vi "CCSaveQueryAsDcmFile.vi"(8 "error in (no error)":errorcluster, 9 "patientID":string="C:\\Users\\Simon\\Dropbox\\Medimatic\\ProjectVerLV2011\\tmp.dcm", 10 "index":i32, 11 "Find":refnum<k24>) -> (0 "error out":errorcluster)   [LabVIEW 2013, in "main.lvlib" / "ClearCanvasLibrary.lvlib"]
uses:
  ClearCanvasLibrary.lvlib
  C:/Users/Simon/SkyDrive/LabView/2013/DM2020/DICOM/ClearCanvasNewBuild/ClearCanvas.Dicom.dll
  ClearCanvasNewBuild/ClearCanvas.Dicom.dll
  Globals/DataPathGlobalVariable.vi
  main.lvlib
  <userlib>/_OpenG.lib/file/file.llb/File Exists - Scalar__ogtk.vi
panel:
  out "DumpString":string
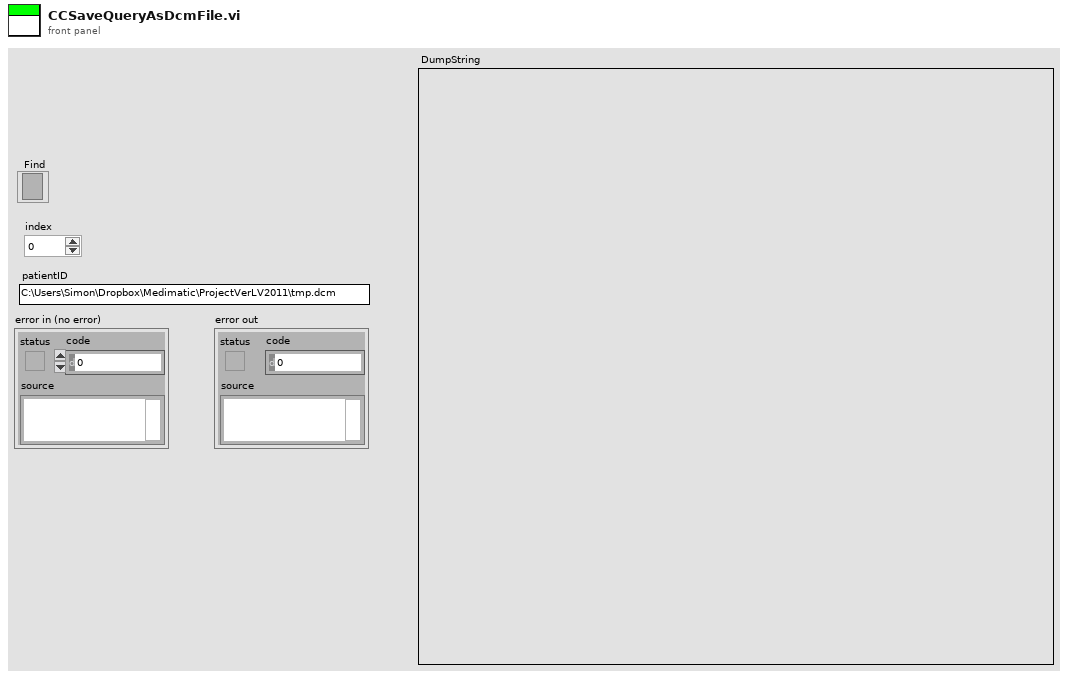
[diagram p1: front panel]
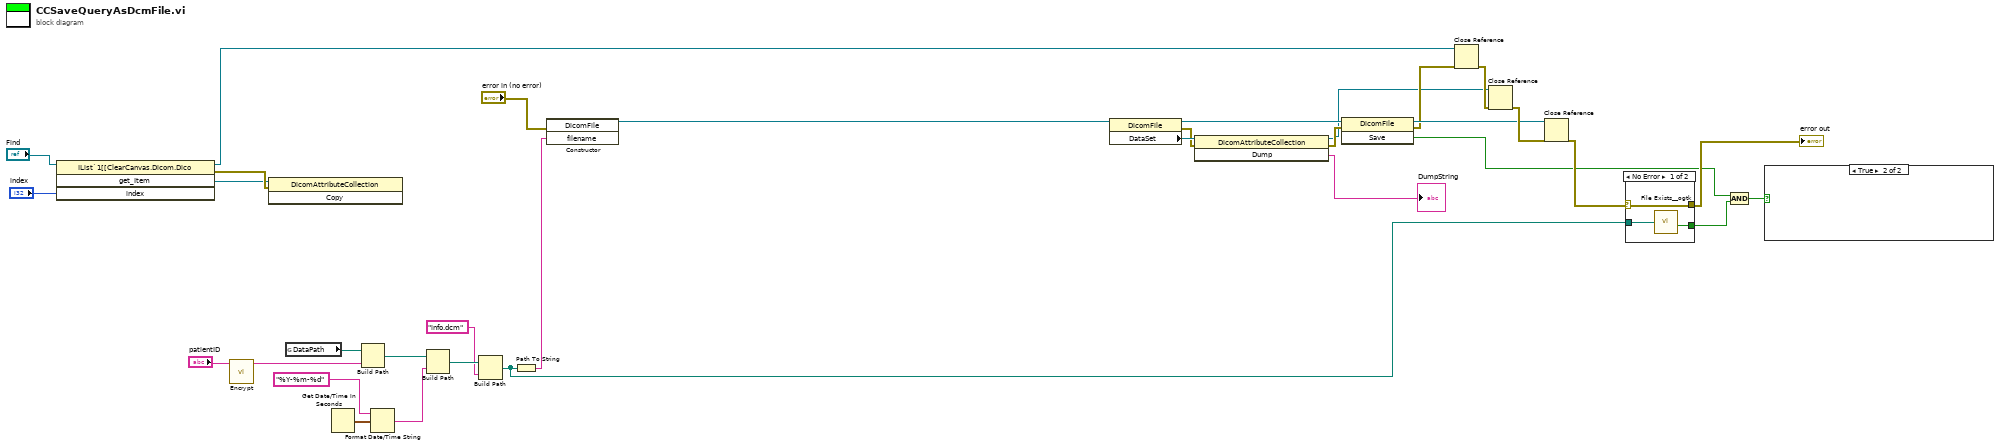
[diagram p0: block diagram]
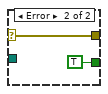
[diagram p2: hidden frame]
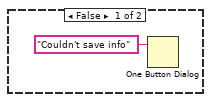
[diagram p3: hidden frame]
diagram:
  n1 = invoke class="IList`1[[ClearCanvas.Dicom.Dico" method="get_Item"(reference="Find", "index"="index") -> (reference out=w2:refnum<k24>, error out=w15:errorcluster, "get_Item"=w1:refnum<k24>)  [unwired: 2 in, 1 out]
  n2 = call "Encrypt.vi"("Input"="patientID") -> ("Output"=w21:string)  [unwired: 10 in]
  n3 = invoke class="DicomAttributeCollection" method="Copy"(reference=w1, error in=w15) -> ()  [unwired: 1 in, 3 out]
  n4 = global read "DataPathGlobalVariable.vi" "DataPath"() -> (w29:path)
  n5 = Get Date/Time In Seconds() -> (seconds since 1Jan1904=w28:timestamp)
  n6 = Build Path(base path=w29, name or relative path=w21) -> (appended path=w26:path)
  n7 = Format Date/Time String(time format string (%c)="%Y-%m-%d", seconds (now)=w28) -> (date/time string=w25:string)  [unwired: 1 in]
  n8 = Build Path(base path=w26, name or relative path=w25) -> (appended path=w24:path)
  n9 = Build Path(base path=w24, name or relative path="info.dcm") -> (appended path=w12:path)
  n10 = Path To String(path=w12) -> (string=w13:string)
  n11 = constructor class="DicomFile"(error in="error in (no error)", "filename"=w13) -> (reference out=w14:refnum<k24>)  [unwired: 2 in, 3 out]
  n12 = property class="DicomFile"(reference=w14) -> (reference out=w11:refnum<k24>, error out=w6:errorcluster, "DataSet"=w7:refnum<k24>)  [unwired: 1 in]
  n13 = invoke class="DicomAttributeCollection" method="Dump"(reference=w7, error in=w6) -> (reference out=w4:refnum<k24>, error out=w5:errorcluster, "Dump"=→"DumpString":string)  [unwired: 1 in]
  n14 = invoke class="DicomFile" method="Save"(reference=w11, error in=w5) -> (reference out=w9:refnum<k24>, error out=w8:errorcluster, "Save"=w10:bool)  [unwired: 1 in]
  n15 = Close Reference(reference=w2, error in (no error)=w8) -> (error out=w31:errorcluster)
  n16 = Close Reference(reference=w4, error in (no error)=w31) -> (error out=w30:errorcluster)
  n17 = Close Reference(reference=w9, error in (no error)=w30) -> (error out=w18:errorcluster)
  n18 = case shown="No Error" w18 {
    selector: w18 -> [w34 w38]
    tunnel: [w36 TRUE ("exists")] -> w19
    tunnel: w12 -> [w35 _]
    tunnel: [w34 w38] -> w17
    frame No Error {
      n19 = call-poly <userlib>:"File Exists__ogtk.vi"("file path"=w35) -> ("exists"=w36:bool)  [unwired: 6 in, 1 out]
    }
    frame Error {
    }
  }
  "error out" <- w17
  n20 = And(x=w10, y=w19) -> (x .and. y?=w20:bool)
  n21 = case shown="True" w20 {
    frame False {
      n22 = One Button Dialog(message="Couldn't save info") -> ()  [unwired: 1 in, 1 out]
    }
    frame True {
    }
  }
